vi "一体站流程质控自动启动.vi"(6 "CODMn量程切换":enum32{"H", "L", "AUTO"}(ring)=enum."AUTO", 8 "总磷量程切换":enum32{"H", "L", "AUTO"}(ring)=enum."AUTO", 9 "总氮量程切换":enum32{"H", "L", "AUTO"}(ring)=enum."AUTO", 10 "氨氮量程切换":enum32{"H", "L", "AUTO"}(ring)=enum."AUTO", 11 "参数":T1={"是否启用仪器"=FALSE, "CODMn"={"启动测量模式"={"测量模式"=enum."水样测量"}, "确定按钮"=TRUE}, "启动模块"={"氨氮"=FALSE, "总磷"=FALSE, "总氮"=FALSE, "CODMn"=FALSE, "CODCr"=FALSE}, "常规启动"=FALSE, "直接启动"=FALSE}) -> ()   [LabVIEW 2016, in "质控单元.lvlib"]
panel:
  out "枚举 2":enum16{"初始化", "采配水启动", "等待", "配水", "排水", "结束"}(ring)
  out "枚举":enum16{"初始化", "采配水启动", "等待", "配水", "排水", "结束"}(ring)
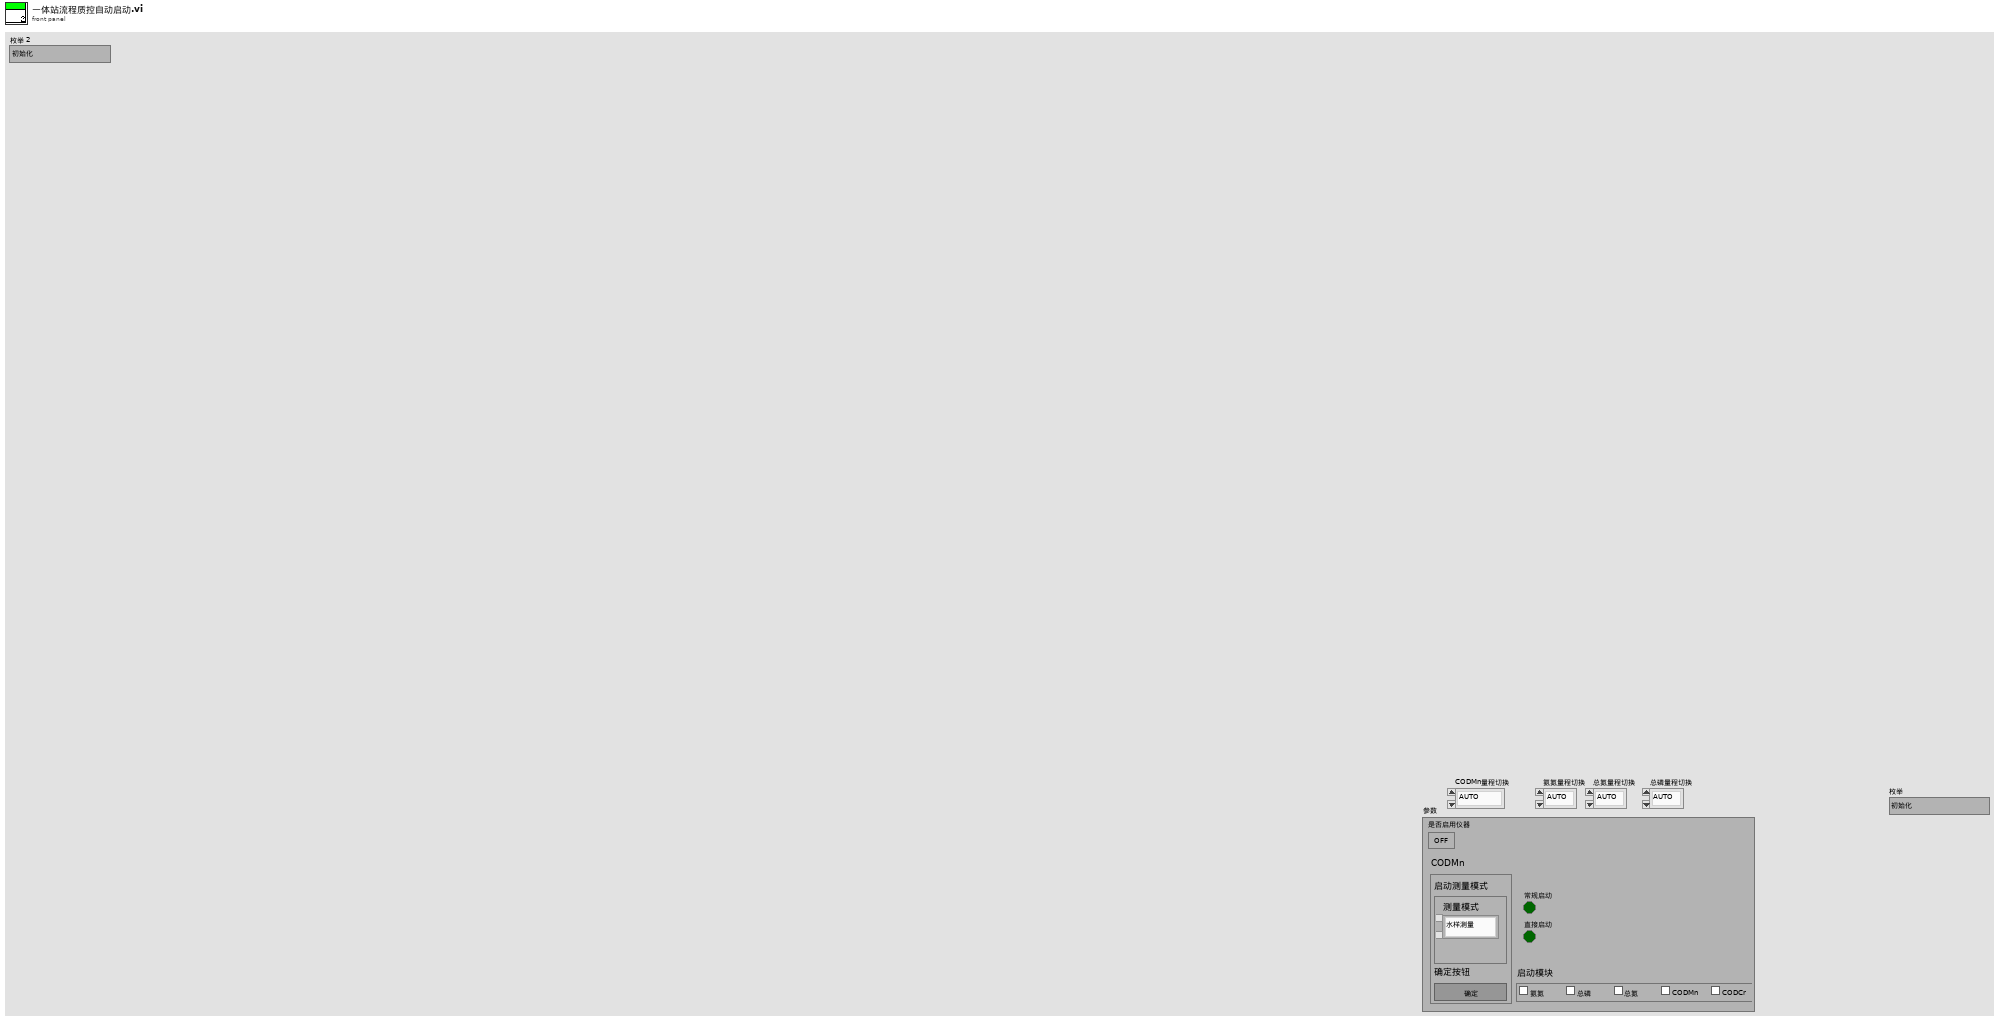
[diagram p1: front panel]
types:
  T1 = cluster{"是否启用仪器":bool, "CODMn":cluster{"启动测量模式":cluster{"测量模式":enum16{"水样测量", "标样核查", "加标回收", "平行样", "校零", "校标"}}, "确定按钮":bool}, "启动模块":cluster{"氨氮":bool, "总磷":bool, "总氮":bool, "CODMn":bool, "CODCr":bool}, "常规启动":bool, "直接启动":bool}
  T2 = cluster{"命令":string, cluster{"starting address":u16, "holding register value":u16}}
  T3 = cluster{"R0":i16, "R1":i16, "R2":i16, "R3":i16, "R4":i16, "R5":i16, "R6":i16, "R7":i16, "R8":i16, "R9":i16, "R10":i16, "R11":i16, "R12":i16, "R13":i16, "R14":i16, "R15":i16, "R16":i16, "R17":i16, "R18":i16, "R19":i16, "R20":i16, "R21":i16, "R22":i16, "R23":i16, "R24":i16, "R25":i16, "R26":i16, "R27":i16, "R28":i16, "R29":i16, "R30":i16, "R31":i16, "R32":i16, "R33":i16, "R34":i16, "R35":i16, "R36":i16, "R37":i16, "R38":i16, "R39":i16, "R40":i16, "R41":i16, "R42":i16, "R43":i16, "R44":i16, "R45":i16, "R46":i16, "R47":i16, "R48":i16, "R49":i16, "R50":i16, "R51":i16, "R52":i16, "R53":i16, "R54":i16, "R55":i16, "R56":i16}
  T4 = enum32{"Bad", "Idle", "Run top level", "Running"}
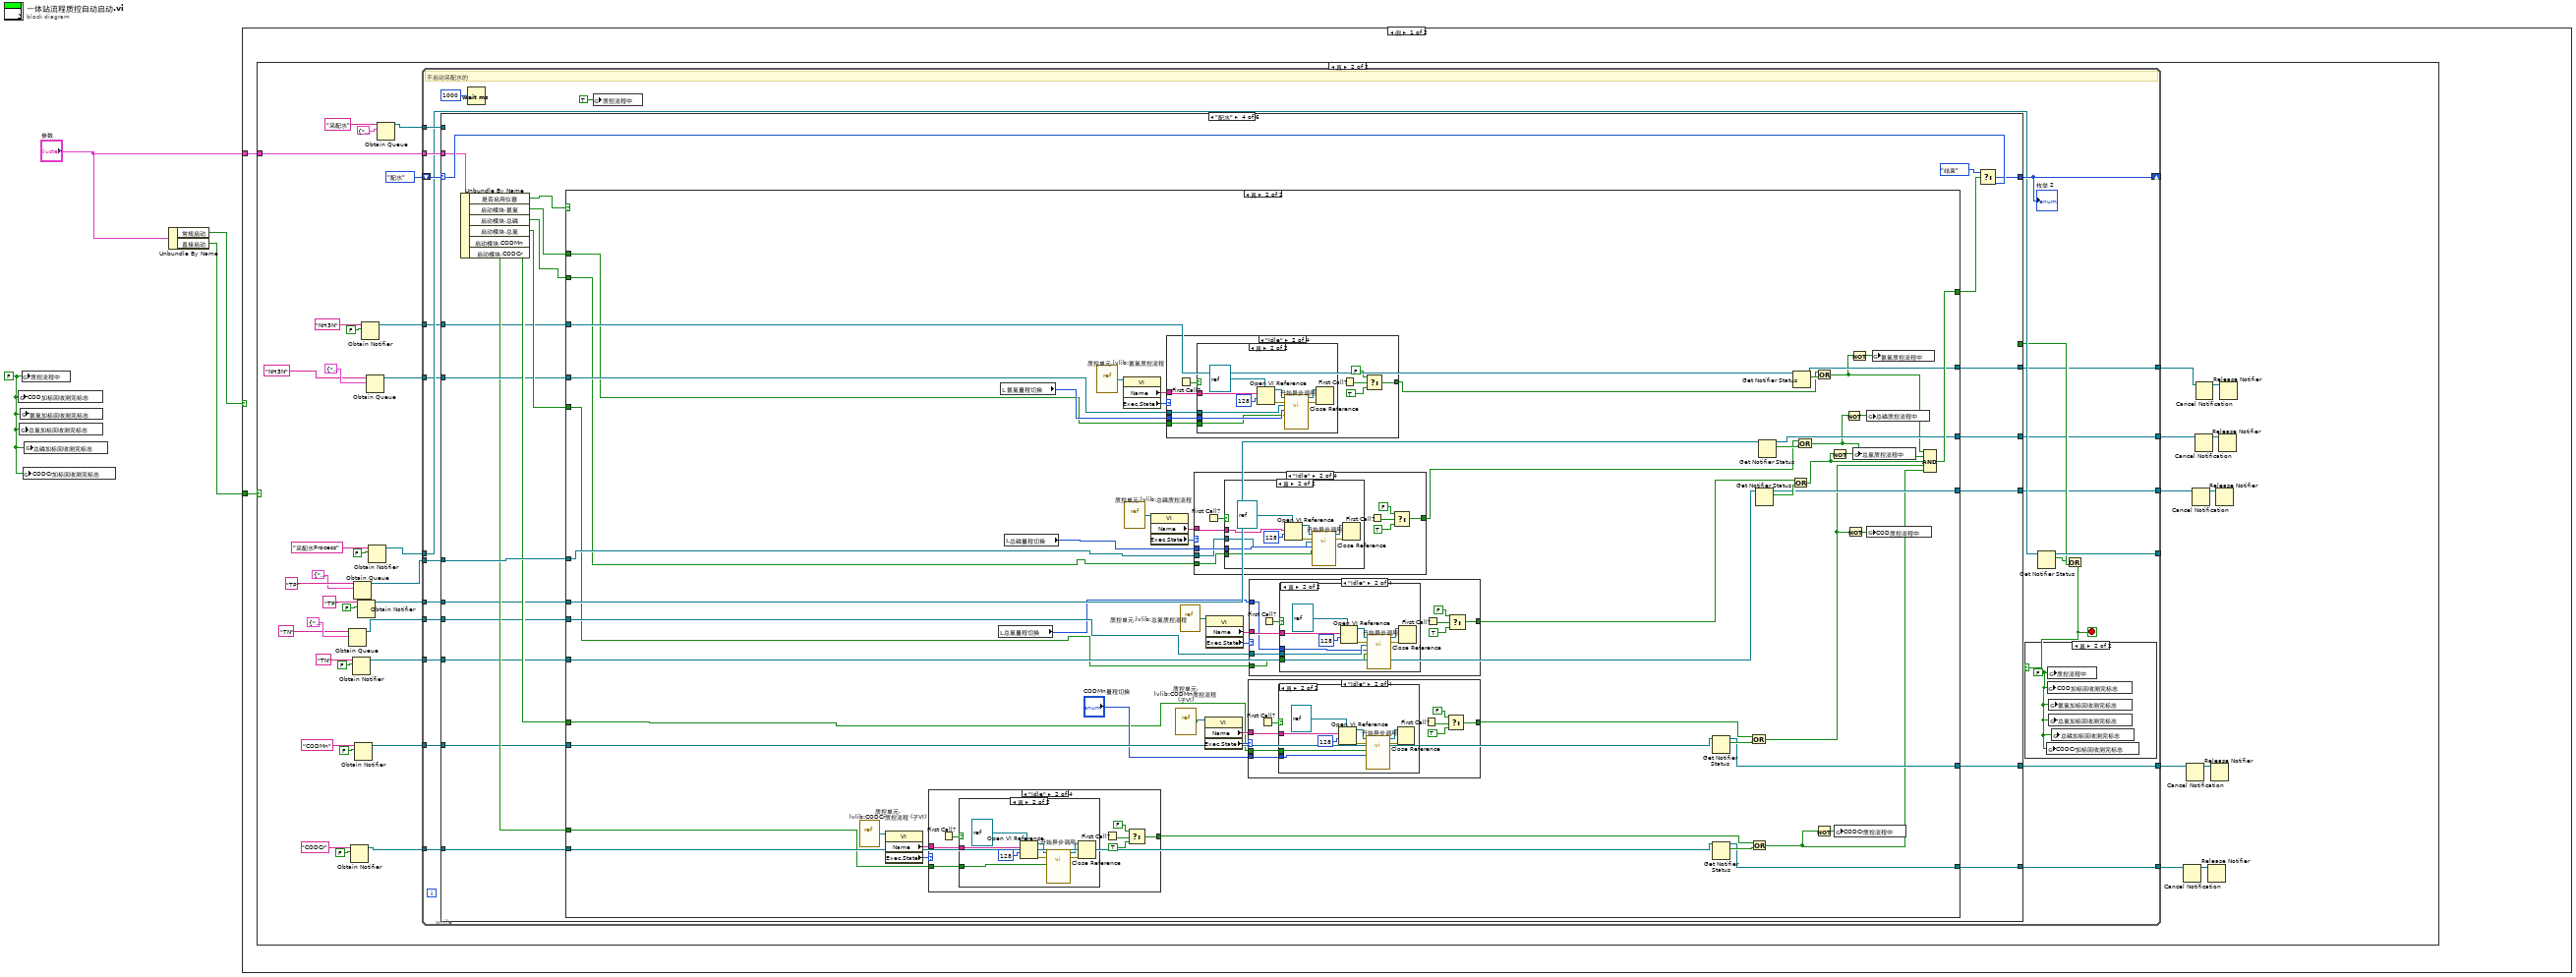
[diagram p0: block diagram]
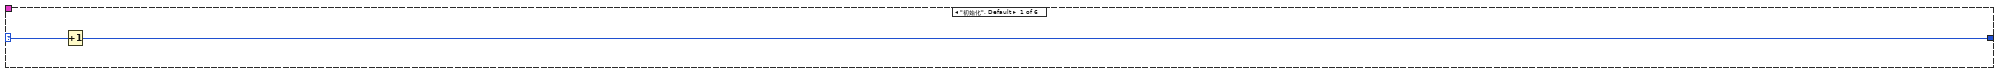
[diagram p4: hidden frame]
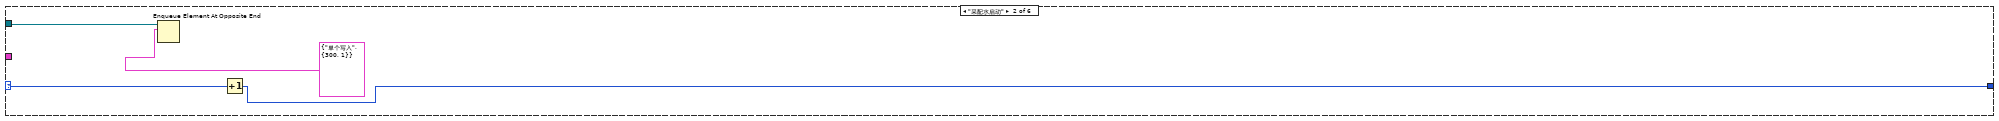
[diagram p5: hidden frame]
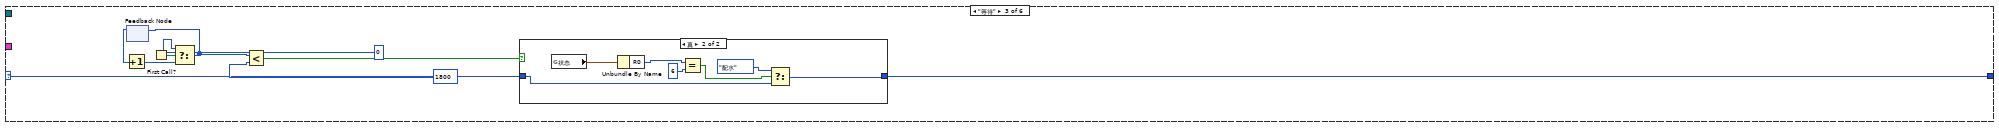
[diagram p6: hidden frame]
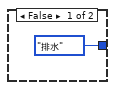
[diagram p7: hidden frame]
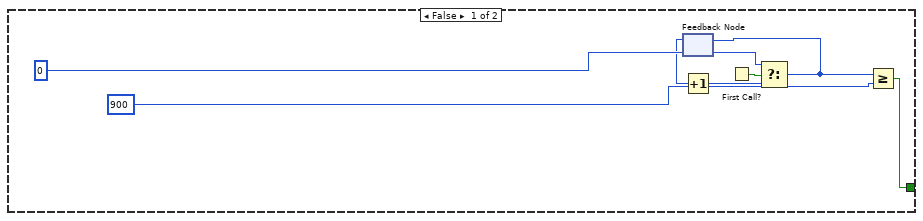
[diagram p8: hidden frame]
diagram:
  w1 = FALSE ("质控流程中")
  n1 = global write "质控测完标志全局 1.vi" "COD加标回收测完标志"(w1) -> ()
  n2 = global write "质控测完标志全局 1.vi" "总氮加标回收测完标志"(w1) -> ()
  n3 = global write "质控测完标志全局 1.vi" "氨氮加标回收测完标志"(w1) -> ()
  n4 = global write "质控测完标志全局 1.vi" "质控流程中"(w1) -> ()
  n5 = global write "质控测完标志全局 1.vi" "CODCr加标回收测完标志"(w1) -> ()
  n6 = global write "质控测完标志全局 1.vi" "总磷加标回收测完标志"(w1) -> ()
  n7 = Unbundle By Name("参数") -> ("常规启动"=w3:bool, "直接启动"=w2:bool)
  n8 = case shown="假" w3 {
    tunnel: "参数" -> [w5 w313]
    tunnel: w2 -> [w6 _]
    frame False {
      n9 = case shown="真" w6 {
        tunnel: w5 -> [_ w47]
        frame False {
        }
        frame True {
          n10 = Obtain Queue(name (unnamed)="TN" ("名称（未命名）"), element data type=cluster{"命令":string, "data":variant} {"命令"="", "data"=variant}) -> (queue out=w32:refnum<queue>)  [unwired: 3 in, 2 out]
          n11 = Obtain Notifier(name (unnamed)="CODCr" ("名称（未命名）"), notification data type=FALSE) -> (notifier out=w9:refnum<notifier>)  [unwired: 2 in, 2 out]
          n12 = Obtain Notifier(name (unnamed)="TN" ("名称（未命名）"), notification data type=FALSE) -> (notifier out=w15:refnum<notifier>)  [unwired: 2 in, 2 out]
          n13 = Obtain Queue(name (unnamed)="TP" ("名称（未命名）"), element data type=cluster{"命令":string, "data":variant} {"命令"="", "data"=variant}) -> (queue out=w38:refnum<queue>)  [unwired: 3 in, 2 out]
          n14 = Obtain Notifier(name (unnamed)="CODMn" ("名称（未命名）"), notification data type=FALSE) -> (notifier out=w12:refnum<notifier>)  [unwired: 2 in, 2 out]
          n15 = Obtain Notifier(name (unnamed)="TP" ("名称（未命名）"), notification data type=FALSE) -> (notifier out=w18:refnum<notifier>)  [unwired: 2 in, 2 out]
          n16 = Obtain Notifier(name (unnamed)="NH3N" ("名称（未命名）"), notification data type=FALSE) -> (notifier out=w21:refnum<notifier>)  [unwired: 2 in, 2 out]
          n17 = Obtain Queue(name (unnamed)="NH3N" ("名称（未命名）"), element data type=cluster{"命令":string, "data":variant} {"命令"="", "data"=variant}) -> (queue out=w35:refnum<queue>)  [unwired: 3 in, 2 out]
          n18 = Obtain Notifier(name (unnamed)="采配水Process" ("名称（未命名）"), notification data type=FALSE) -> (notifier out=w41:refnum<notifier>)  [unwired: 2 in, 2 out]
          n19 = Obtain Queue(name (unnamed)="采配水" ("名称（未命名）"), element data type=cluster{"命令":string, "数据":variant} {"命令"="", "数据"=variant}) -> (queue out=w44:refnum<queue>)  [unwired: 3 in, 2 out]
          n20 = while {
            tunnel: w44 -> [w72]
            shift-right: [w70] -> _
            shift-left: enum16{"初始化", "采配水启动", "等待", "配水", "排水", "结束"}."配水" ("枚举") -> [w71]
            tunnel: w38 -> [w68]
            tunnel: w47 -> [w67]
            tunnel: w41 -> [w66]
            tunnel: [w65] -> _
            tunnel: w35 -> [w62]
            tunnel: w32 -> [w59]
            tunnel: w21 -> [w58]
            tunnel: [w57] -> w19
            tunnel: w18 -> [w56]
            tunnel: [w55] -> w16
            tunnel: w15 -> [w54]
            tunnel: [w53] -> w13
            tunnel: w12 -> [w52]
            tunnel: [w51] -> w10
            tunnel: w9 -> [w50]
            tunnel: [w49] -> w7
            stop <- w61 stop-if-true
            # "不启动采配水的"
            n21 = case shown="\"配水\"" w71 {
              selector: w71 -> [w75 w77 w86 w119 w276 w281]
              tunnel: w72 -> [_ w78 _ _ w277 _]
              tunnel: [w74 w76 w85 w118 w275 w280] -> w70
              tunnel: [_ _ _ _ _ TRUE] -> w64
              tunnel: w68 -> [_ _ _ w117 _ _]
              tunnel: w67 -> [_ _ _ w114 _ _]
              tunnel: w62 -> [_ _ _ w109 _ _]
              tunnel: w59 -> [_ _ _ w107 _ _]
              tunnel: w58 -> [_ _ _ w106 _ _]
              tunnel: [_ _ _ w105 _ _] -> w57
              tunnel: w56 -> [_ _ _ w104 _ _]
              tunnel: [_ _ _ w103 _ _] -> w55
              tunnel: w54 -> [_ _ _ w102 _ _]
              tunnel: [_ _ _ w101 _ _] -> w53
              tunnel: w52 -> [_ _ _ w100 _ _]
              tunnel: [_ _ _ w99 _ _] -> w51
              tunnel: w50 -> [_ _ _ w98 _ _]
              tunnel: [_ _ _ w97 _ _] -> w49
              frame "初始化", Default {
                n22 = Increment(x=w75) -> (x+1=w74:enum16{"初始化", "采配水启动", "等待", "配水", "排水", "结束"})
              }
              frame "采配水启动" {
                n23 = Enqueue Element At Opposite End(queue=w78, element=T2 {"命令"="单个写入", {"starting address"=300, "holding register value"=1}} ("元素")) -> ()  [unwired: 2 in, 3 out]
                n24 = Increment(x=w77) -> (x+1=w76:enum16{"初始化", "采配水启动", "等待", "配水", "排水", "结束"})
              }
              frame "等待" {
                n25 = feedback #1() -> (w82:i32)  [unwired: 1 in]
                n26 = Increment(x=w82) -> (x+1=w81:i32)
                n27 = First Call?() -> (First Call?: T/F=w83:bool)
                n28 = Select(t=0, s=w83, f=w81) -> (s? t:f=w80:i32)
                n29 = feedback-in #1(w80) -> ()
                n30 = Less?(x=w80, y=1800) -> (x < y?=w87:bool)
                n31 = case shown="真" w87 {
                  tunnel: w86 -> [_ w92]
                  tunnel: [enum16{"初始化", "采配水启动", "等待", "配水", "排水", "结束"}."排水" ("枚举") w91] -> w85
                  frame False {
                  }
                  frame True {
                    n32 = global read "与采配水交互全局.vi" "状态"() -> (w90:T3)
                    n33 = Unbundle By Name(w90) -> ("R0"=w96:i16)
                    n34 = Equal?(x=w96, y=i16 6) -> (x = y?=w94:bool)
                    n35 = Select(t=enum16{"初始化", "采配水启动", "等待", "配水", "排水", "结束"}."配水" ("枚举"), s=w94, f=w92) -> (s? t:f=w91:enum16{"初始化", "采配水启动", "等待", "配水", "排水", "结束"})
                  }
                }
              }
              frame "配水" {
                n36 = Unbundle By Name(w114) -> ("是否启用仪器"=w116:bool, "启动模块.氨氮"=w112:bool, "启动模块.总磷"=w113:bool, "启动模块.总氮"=w110:bool, "启动模块.CODMn"=w111:bool, "启动模块.CODCr"=w108:bool)
                n37 = case shown="真" w116 {
                  tunnel: w117 -> [_ w149]
                  tunnel: [w121 w185] -> w115
                  tunnel: w113 -> [_ w147]
                  tunnel: w112 -> [_ w154]
                  tunnel: w111 -> [_ w136]
                  tunnel: w110 -> [_ w141]
                  tunnel: w109 -> [_ w156]
                  tunnel: w108 -> [_ w129]
                  tunnel: w107 -> [_ w143]
                  tunnel: w106 -> [_ w183]
                  tunnel: [_ w182] -> w105
                  tunnel: w104 -> [_ w180]
                  tunnel: [_ w179] -> w103
                  tunnel: w102 -> [_ w177]
                  tunnel: [_ w176] -> w101
                  tunnel: w100 -> [_ w174]
                  tunnel: [_ w173] -> w99
                  tunnel: w98 -> [_ w171]
                  tunnel: [_ w170] -> w97
                  frame False {
                    n38 = feedback #2() -> (w125:i32)  [unwired: 1 in]
                    n39 = Increment(x=w125) -> (x+1=w124:i32)
                    n40 = First Call?() -> (First Call?: T/F=w126:bool)
                    n41 = Select(t=0, s=w126, f=w124) -> (s? t:f=w122:i32)
                    n42 = feedback-in #2(w122) -> ()
                    n43 = Greater Or Equal?(x=w122, y=900) -> (x >= y?=w121:bool)
                  }
                  frame True {
                    n44 = vi-ref "质控单元.lvlib:CODCr质控流程 (子VI).vi"() -> (w131:refnum<vi>)
                    n45 = property class="VI"(reference=w131) -> ("Name"=w132:string, "Exec.State"=w130:T4)  [unwired: 1 in, 2 out]
                    n46 = case shown="\"Idle\"" w130 {
                      tunnel: w132 -> [_ w192 _ _]
                      tunnel: [_ w187 _ _] -> w128
                      tunnel: w129 -> [_ w186 _ _]
                      frame "Bad", Default {
                      }
                      frame "Idle" {
                        n47 = First Call?() -> (First Call?: T/F=w191:bool)
                        n48 = case shown="真" w191 {
                          tunnel: w192 -> [_ w199]
                          tunnel: w186 -> [_ w193]
                          frame False {
                          }
                          frame True {
                            n49 = Open VI Reference(type specifier VI Refnum (for type only)=refnum<vi> refnum ("类型说明符VI引用句柄（仅用于类型）"), vi path=w199, options=128 ("选项")) -> (vi reference=w200:refnum<vi>, error out=w196:errorcluster)  [unwired: 3 in]
                            n50 = call-by-ref "开始异步调用"(reference=w200, error in=w196, "CODCr"=w193) -> (reference out=w198:refnum<vi>, error out=w197:errorcluster)  [unwired: 9 in, 1 out]
                            n51 = Close Reference(reference=w198, error in (no error)=w197) -> ()  [unwired: 1 out]
                          }
                        }
                        n52 = First Call?() -> (First Call?: T/F=w190:bool)
                        n53 = Select(t=FALSE, s=w190, f=TRUE) -> (s? t:f=w187:bool)
                      }
                      frame "Run top level" {
                      }
                      frame "Running" {
                      }
                    }
                    n54 = local read "总氮量程切换"() -> (w142:enum32{"H", "L", "AUTO"})
                    n55 = local read "氨氮量程切换"() -> (w155:enum32{"H", "L", "AUTO"})
                    n56 = local read "总磷量程切换"() -> (w148:enum32{"H", "L", "AUTO"})
                    n57 = vi-ref "质控单元.lvlib:氨氮质控流程.vi"() -> (w158:refnum<vi>)
                    n58 = property class="VI"(reference=w158) -> ("Name"=w159:string, "Exec.State"=w157:T4)  [unwired: 1 in, 2 out]
                    n59 = vi-ref "质控单元.lvlib:总磷质控流程.vi"() -> (w151:refnum<vi>)
                    n60 = property class="VI"(reference=w151) -> ("Name"=w150:string, "Exec.State"=w152:T4)  [unwired: 1 in, 2 out]
                    n61 = case shown="\"Idle\"" w157 {
                      tunnel: w159 -> [_ w264 _ _]
                      tunnel: [_ w259 _ _] -> w153
                      tunnel: w156 -> [_ w258 _ _]
                      tunnel: w155 -> [_ w257 _ _]
                      tunnel: w154 -> [_ w256 _ _]
                      frame "Bad", Default {
                      }
                      frame "Idle" {
                        n62 = First Call?() -> (First Call?: T/F=w263:bool)
                        n63 = case shown="真" w263 {
                          tunnel: w264 -> [_ w273]
                          tunnel: w258 -> [_ w267]
                          tunnel: w257 -> [_ w266]
                          tunnel: w256 -> [_ w265]
                          frame False {
                          }
                          frame True {
                            n64 = Open VI Reference(type specifier VI Refnum (for type only)=refnum<vi> refnum ("类型说明符VI引用句柄（仅用于类型）"), vi path=w273, options=128 ("选项")) -> (vi reference=w274:refnum<vi>, error out=w270:errorcluster)  [unwired: 3 in]
                            n65 = call-by-ref "开始异步调用"(reference=w274, error in=w270, "队列输入NH3"=w267, "氨氮"=w265, "氨氮量程切换"=w266) -> (reference out=w272:refnum<vi>, error out=w271:errorcluster)  [unwired: 7 in, 1 out]
                            n66 = Close Reference(reference=w272, error in (no error)=w271) -> ()  [unwired: 1 out]
                          }
                        }
                        n67 = First Call?() -> (First Call?: T/F=w262:bool)
                        n68 = Select(t=FALSE, s=w262, f=TRUE) -> (s? t:f=w259:bool)
                      }
                      frame "Run top level" {
                      }
                      frame "Running" {
                      }
                    }
                    n69 = vi-ref "质控单元.lvlib:CODMn质控流程 (子VI).vi"() -> (w139:refnum<vi>)
                    n70 = vi-ref "质控单元.lvlib:总氮质控流程.vi"() -> (w145:refnum<vi>)
                    n71 = case shown="\"Idle\"" w152 {
                      tunnel: w150 -> [_ w245 _ _]
                      tunnel: [_ w240 _ _] -> w134
                      tunnel: w148 -> [_ w239 _ _]
                      tunnel: w147 -> [_ w238 _ _]
                      tunnel: w149 -> [_ w237 _ _]
                      frame "Bad", Default {
                      }
                      frame "Idle" {
                        n72 = First Call?() -> (First Call?: T/F=w244:bool)
                        n73 = case shown="真" w244 {
                          tunnel: w245 -> [_ w246]
                          tunnel: w239 -> [_ w254]
                          tunnel: w238 -> [_ w252]
                          tunnel: w237 -> [_ w251]
                          frame False {
                          }
                          frame True {
                            n74 = Open VI Reference(type specifier VI Refnum (for type only)=refnum<vi> refnum ("类型说明符VI引用句柄（仅用于类型）"), vi path=w246, options=128 ("选项")) -> (vi reference=w250:refnum<vi>, error out=w249:errorcluster)  [unwired: 3 in]
                            n75 = call-by-ref "开始异步调用"(reference=w250, error in=w249, "队列输入TP"=w251, "总磷"=w252, "总磷量程切换"=w254) -> (reference out=w248:refnum<vi>, error out=w247:errorcluster)  [unwired: 7 in, 1 out]
                            n76 = Close Reference(reference=w248, error in (no error)=w247) -> ()  [unwired: 1 out]
                          }
                        }
                        n77 = First Call?() -> (First Call?: T/F=w243:bool)
                        n78 = Select(t=FALSE, s=w243, f=TRUE) -> (s? t:f=w240:bool)
                      }
                      frame "Run top level" {
                      }
                      frame "Running" {
                      }
                    }
                    n79 = property class="VI"(reference=w139) -> ("Name"=w138:string, "Exec.State"=w140:T4)  [unwired: 1 in, 2 out]
                    n80 = property class="VI"(reference=w145) -> ("Name"=w146:string, "Exec.State"=w144:T4)  [unwired: 1 in, 2 out]
                    n81 = case shown="\"Idle\"" w140 {
                      tunnel: w138 -> [_ w208 _ _]
                      tunnel: [_ w203 _ _] -> w135
                      tunnel: w136 -> [_ w202 _ _]
                      tunnel: "CODMn量程切换" -> [_ w201 _ _]
                      frame "Bad", Default {
                      }
                      frame "Idle" {
                        n82 = First Call?() -> (First Call?: T/F=w207:bool)
                        n83 = case shown="真" w207 {
                          tunnel: w208 -> [_ w216]
                          tunnel: w202 -> [_ w210]
                          tunnel: w201 -> [_ w209]
                          frame False {
                          }
                          frame True {
                            n84 = Open VI Reference(type specifier VI Refnum (for type only)=refnum<vi> refnum ("类型说明符VI引用句柄（仅用于类型）"), vi path=w216, options=128 ("选项")) -> (vi reference=w217:refnum<vi>, error out=w213:errorcluster)  [unwired: 3 in]
                            n85 = call-by-ref "开始异步调用"(reference=w217, error in=w213, "CODMn量程切换"=w209, "CODMn"=w210) -> (reference out=w215:refnum<vi>, error out=w214:errorcluster)  [unwired: 8 in, 1 out]
                            n86 = Close Reference(reference=w215, error in (no error)=w214) -> ()  [unwired: 1 out]
                          }
                        }
                        n87 = First Call?() -> (First Call?: T/F=w206:bool)
                        n88 = Select(t=FALSE, s=w206, f=TRUE) -> (s? t:f=w203:bool)
                      }
                      frame "Run top level" {
                      }
                      frame "Running" {
                      }
                    }
                    n89 = case shown="\"Idle\"" w144 {
                      tunnel: w146 -> [_ w226 _ _]
                      tunnel: [_ w221 _ _] -> w133
                      tunnel: w143 -> [_ w220 _ _]
                      tunnel: w142 -> [_ w219 _ _]
                      tunnel: w141 -> [_ w218 _ _]
                      frame "Bad", Default {
                      }
                      frame "Idle" {
                        n90 = First Call?() -> (First Call?: T/F=w225:bool)
                        n91 = case shown="真" w225 {
                          tunnel: w226 -> [_ w236]
                          tunnel: w220 -> [_ w229]
                          tunnel: w219 -> [_ w228]
                          tunnel: w218 -> [_ w227]
                          frame False {
                          }
                          frame True {
                            n92 = Open VI Reference(type specifier VI Refnum (for type only)=refnum<vi> refnum ("类型说明符VI引用句柄（仅用于类型）"), vi path=w236, options=128 ("选项")) -> (vi reference=w231:refnum<vi>, error out=w230:errorcluster)  [unwired: 3 in]
                            n93 = call-by-ref "开始异步调用"(reference=w231, error in=w230, "队列输入TN"=w229, "总氮"=w227, "总氮量程切换"=w228) -> (reference out=w235:refnum<vi>, error out=w234:errorcluster)  [unwired: 7 in, 1 out]
                            n94 = Close Reference(reference=w235, error in (no error)=w234) -> ()  [unwired: 1 out]
                          }
                        }
                        n95 = First Call?() -> (First Call?: T/F=w224:bool)
                        n96 = Select(t=FALSE, s=w224, f=TRUE) -> (s? t:f=w221:bool)
                      }
                      frame "Run top level" {
                      }
                      frame "Running" {
                      }
                    }
                    n97 = Get Notifier Status(notifier=w174) -> (notifier out=w173:refnum<notifier>, current notification=w175:bool)  [unwired: 1 in, 3 out]
                    n98 = Get Notifier Status(notifier=w171) -> (notifier out=w170:refnum<notifier>, current notification=w172:bool)  [unwired: 1 in, 3 out]
                    n99 = Or(x=w135, y=w175) -> (x .or. y?=w162:bool)
                    n100 = Or(x=w128, y=w172) -> (x .or. y?=w160:bool)
                    n101 = Get Notifier Status(notifier=w177) -> (notifier out=w176:refnum<notifier>, current notification=w178:bool)  [unwired: 1 in, 3 out]
                    n102 = Get Notifier Status(notifier=w180) -> (notifier out=w179:refnum<notifier>, current notification=w181:bool)  [unwired: 1 in, 3 out]
                    n103 = Or(x=w133, y=w178) -> (x .or. y?=w164:bool)
                    n104 = Get Notifier Status(notifier=w183) -> (notifier out=w182:refnum<notifier>, current notification=w184:bool)  [unwired: 1 in, 3 out]
                    n105 = Or(x=w134, y=w181) -> (x .or. y?=w166:bool)
                    n106 = Not(x=w160) -> (.not. x?=w161:bool)
                    n107 = Or(x=w153, y=w184) -> (x .or. y?=w168:bool)
                    n108 = Not(x=w164) -> (.not. x?=w165:bool)
                    n109 = global write "质控测完标志全局 1.vi" "CODCr质控流程中"(w161) -> ()
                    n110 = Not(x=w166) -> (.not. x?=w167:bool)
                    n111 = Not(x=w162) -> (.not. x?=w163:bool)
                    n112 = Not(x=w168) -> (.not. x?=w169:bool)
                    n113 = global write "质控测完标志全局 1.vi" "总氮质控流程中"(w165) -> ()
                    n114 = global write "质控测完标志全局 1.vi" "总磷质控流程中"(w167) -> ()
                    n115 = global write "质控测完标志全局 1.vi" "COD质控流程中"(w163) -> ()
                    n116 = global write "质控测完标志全局 1.vi" "氨氮质控流程中"(w169) -> ()
                    n117 = Compound Arithmetic op=AND ("复合运算")(w168, w166, w164, w162, w160) -> (w185:bool)
                  }
                }
                n118 = Select(t=enum16{"初始化", "采配水启动", "等待", "配水", "排水", "结束"}."结束" ("枚举"), s=w115, f=w119) -> (s? t:f=w118:enum16{"初始化", "采配水启动", "等待", "配水", "排水", "结束"})
              }
              frame "排水" {
                n119 = Enqueue Element At Opposite End(queue=w277, element=T2 {"命令"="单个写入", {"starting address"=303, "holding register value"=1}} ("元素")) -> ()  [unwired: 2 in, 3 out]
                n120 = Increment(x=w276) -> (x+1=w275:enum16{"初始化", "采配水启动", "等待", "配水", "排水", "结束"})
              }
              frame "结束" {
                n121 = Increment(x=w281) -> (x+1=w280:enum16{"初始化", "采配水启动", "等待", "配水", "排水", "结束"})
              }
            }
            "枚举 2" <- w70
            n122 = Wait (ms)(milliseconds to wait=u32 1000 ("等待时间（毫秒）")) -> ()  [unwired: 1 out]
            n123 = global write "质控测完标志全局 1.vi" "质控流程中"(TRUE ("质控流程中")) -> ()
            n124 = Get Notifier Status(notifier=w66) -> (notifier out=w65:refnum<notifier>, current notification=w63:bool)  [unwired: 1 in, 3 out]
            n125 = Or(x=w63, y=w64) -> (x .or. y?=w61:bool)
            n126 = case shown="真" w61 {
              frame False {
              }
              frame True {
                w73 = FALSE ("质控流程中")
                n127 = global write "质控测完标志全局 1.vi" "CODCr加标回收测完标志"(w73) -> ()
                n128 = global write "质控测完标志全局 1.vi" "COD加标回收测完标志"(w73) -> ()
                n129 = global write "质控测完标志全局 1.vi" "质控流程中"(w73) -> ()
                n130 = global write "质控测完标志全局 1.vi" "总氮加标回收测完标志"(w73) -> ()
                n131 = global write "质控测完标志全局 1.vi" "氨氮加标回收测完标志"(w73) -> ()
                n132 = global write "质控测完标志全局 1.vi" "总磷加标回收测完标志"(w73) -> ()
              }
            }
          }
          n133 = Cancel Notification(0:w7) -> (8:w8:refnum<notifier>)  [unwired: 1 in, 2 out]
          n134 = Cancel Notification(0:w10) -> (8:w11:refnum<notifier>)  [unwired: 1 in, 2 out]
          n135 = Cancel Notification(0:w13) -> (8:w14:refnum<notifier>)  [unwired: 1 in, 2 out]
          n136 = Cancel Notification(0:w16) -> (8:w17:refnum<notifier>)  [unwired: 1 in, 2 out]
          n137 = Cancel Notification(0:w19) -> (8:w20:refnum<notifier>)  [unwired: 1 in, 2 out]
          n138 = Release Notifier(notifier=w8) -> ()  [unwired: 2 in, 3 out]
          n139 = Release Notifier(notifier=w11) -> ()  [unwired: 2 in, 3 out]
          n140 = Release Notifier(notifier=w14) -> ()  [unwired: 2 in, 3 out]
          n141 = Release Notifier(notifier=w17) -> ()  [unwired: 2 in, 3 out]
          n142 = Release Notifier(notifier=w20) -> ()  [unwired: 2 in, 3 out]
        }
      }
    }
    frame True {
      n143 = Obtain Notifier(name (unnamed)="采配水Process" ("名称（未命名）"), notification data type=FALSE) -> (notifier out=w316:refnum<notifier>)  [unwired: 2 in, 2 out]
      n144 = Obtain Notifier(name (unnamed)="TN" ("名称（未命名）"), notification data type=FALSE) -> (notifier out=w298:refnum<notifier>)  [unwired: 2 in, 2 out]
      n145 = Obtain Notifier(name (unnamed)="CODCr" ("名称（未命名）"), notification data type=FALSE) -> (notifier out=w292:refnum<notifier>)  [unwired: 2 in, 2 out]
      n146 = Obtain Queue(name (unnamed)="TN" ("名称（未命名）"), element data type=cluster{"命令":string, "data":variant} {"命令"="", "data"=variant}) -> (queue out=w310:refnum<queue>)  [unwired: 3 in, 2 out]
      n147 = Obtain Notifier(name (unnamed)="CODMn" ("名称（未命名）"), notification data type=FALSE) -> (notifier out=w293:refnum<notifier>)  [unwired: 2 in, 2 out]
      n148 = Obtain Notifier(name (unnamed)="TP" ("名称（未命名）"), notification data type=FALSE) -> (notifier out=w299:refnum<notifier>)  [unwired: 2 in, 2 out]
      n149 = Obtain Queue(name (unnamed)="TP" ("名称（未命名）"), element data type=cluster{"命令":string, "data":variant} {"命令"="", "data"=variant}) -> (queue out=w319:refnum<queue>)  [unwired: 3 in, 2 out]
      n150 = Obtain Queue(name (unnamed)="NH3N" ("名称（未命名）"), element data type=cluster{"命令":string, "data":variant} {"命令"="", "data"=variant}) -> (queue out=w305:refnum<queue>)  [unwired: 3 in, 2 out]
      n151 = Obtain Notifier(name (unnamed)="NH3N" ("名称（未命名）"), notification data type=FALSE) -> (notifier out=w304:refnum<notifier>)  [unwired: 2 in, 2 out]
      n152 = Obtain Queue(name (unnamed)="采配水" ("名称（未命名）"), element data type=cluster{"命令":string, "数据":variant} {"命令"="", "数据"=variant}) -> (queue out=w323:refnum<queue>)  [unwired: 3 in, 2 out]
      n153 = while {
        tunnel: w323 -> [w349]
        shift-right: [w347] -> _
        shift-left: enum16{"初始化", "采配水启动", "等待", "配水", "排水", "结束"}."初始化" ("枚举") -> [w348]
        tunnel: w319 -> [w345]
        tunnel: w313 -> [w344]
        tunnel: w316 -> [w343]
        tunnel: [w342] -> w315
        tunnel: w310 -> [w337]
        tunnel: w305 -> [w336]
        tunnel: w304 -> [w335]
        tunnel: w299 -> [w334]
        tunnel: w298 -> [w333]
        tunnel: w293 -> [w332]
        tunnel: w292 -> [w331]
        tunnel: [w330] -> w290
        tunnel: [w329] -> w288
        tunnel: [w328] -> w286
        tunnel: [w327] -> w284
        tunnel: [w326] -> w282
        stop <- w339 stop-if-true
        # "启动采配水的"
        n154 = case shown="\"配水\"" w348 {
          selector: w348 -> [w352 w354 w363 w396 w548 w553]
          tunnel: w349 -> [_ w355 _ _ w549 _]
          tunnel: [w351 w353 w362 w395 w547 w552] -> w347
          tunnel: [_ _ _ _ _ TRUE] -> w341
          tunnel: w345 -> [_ _ _ w394 _ _]
          tunnel: w344 -> [_ _ _ w391 _ _]
          tunnel: w337 -> [_ _ _ w385 _ _]
          tunnel: w336 -> [_ _ _ w384 _ _]
          tunnel: w335 -> [_ _ _ w383 _ _]
          tunnel: w334 -> [_ _ _ w382 _ _]
          tunnel: w333 -> [_ _ _ w381 _ _]
          tunnel: w332 -> [_ _ _ w380 _ _]
          tunnel: w331 -> [_ _ _ w379 _ _]
          tunnel: [_ _ _ w378 _ _] -> w330
          tunnel: [_ _ _ w377 _ _] -> w329
          tunnel: [_ _ _ w376 _ _] -> w328
          tunnel: [_ _ _ w375 _ _] -> w327
          tunnel: [_ _ _ w374 _ _] -> w326
          frame "初始化", Default {
            n155 = Increment(x=w352) -> (x+1=w351:enum16{"初始化", "采配水启动", "等待", "配水", "排水", "结束"})
          }
          frame "采配水启动" {
            n156 = Enqueue Element At Opposite End(queue=w355, element=T2 {"命令"="单个写入", {"starting address"=300, "holding register value"=3}} ("元素")) -> ()  [unwired: 2 in, 3 out]
            n157 = Increment(x=w354) -> (x+1=w353:enum16{"初始化", "采配水启动", "等待", "配水", "排水", "结束"})
          }
          frame "等待" {
            n158 = feedback #3() -> (w359:i32)  [unwired: 1 in]
            n159 = Increment(x=w359) -> (x+1=w358:i32)
            n160 = First Call?() -> (First Call?: T/F=w360:bool)
            n161 = Select(t=0, s=w360, f=w358) -> (s? t:f=w357:i32)
            n162 = feedback-in #3(w357) -> ()
            n163 = Less?(x=w357, y=1800) -> (x < y?=w364:bool)
            n164 = case shown="真" w364 {
              tunnel: w363 -> [_ w369]
              tunnel: [enum16{"初始化", "采配水启动", "等待", "配水", "排水", "结束"}."排水" ("枚举") w368] -> w362
              frame False {
              }
              frame True {
                n165 = global read "与采配水交互全局.vi" "状态"() -> (w367:T3)
                n166 = Unbundle By Name(w367) -> ("R0"=w373:i16)
                n167 = Equal?(x=w373, y=i16 6) -> (x = y?=w371:bool)
                n168 = Select(t=enum16{"初始化", "采配水启动", "等待", "配水", "排水", "结束"}."配水" ("枚举"), s=w371, f=w369) -> (s? t:f=w368:enum16{"初始化", "采配水启动", "等待", "配水", "排水", "结束"})
              }
            }
          }
          frame "配水" {
            (unwired) cluster{"命令":string, "data":variant} {"命令"="启动", "data"=variant(cluster{"站号":u16, "控制命令输出":u16[]} {"站号"=1, "控制命令输出"=[256, 0]})} ("元素")
            n169 = Unbundle By Name(w391) -> ("是否启用仪器"=w393:bool, "启动模块.氨氮"=w389:bool, "启动模块.总磷"=w390:bool, "启动模块.总氮"=w387:bool, "启动模块.CODMn"=w388:bool, "启动模块.CODCr"=w386:bool)
            n170 = case shown="真" w393 {
              tunnel: w394 -> [_ w414]
              tunnel: [w398 w457] -> w392
              tunnel: w390 -> [_ w415]
              tunnel: w389 -> [_ w431]
              tunnel: w388 -> [_ w409]
              tunnel: w387 -> [_ w411]
              tunnel: w384 -> [_ w433]
              tunnel: w386 -> [_ w406]
              tunnel: w385 -> [_ w413]
              tunnel: w383 -> [_ w454]
              tunnel: w382 -> [_ w451]
              tunnel: w381 -> [_ w449]
              tunnel: w380 -> [_ w443]
              tunnel: w379 -> [_ w442]
              tunnel: [_ w441] -> w378
              tunnel: [_ w440] -> w377
              tunnel: [_ w439] -> w376
              tunnel: [_ w438] -> w375
              tunnel: [_ w437] -> w374
              frame False {
                n171 = feedback #4() -> (w402:i32)  [unwired: 1 in]
                n172 = Increment(x=w402) -> (x+1=w401:i32)
                n173 = First Call?() -> (First Call?: T/F=w403:bool)
                n174 = Select(t=0, s=w403, f=w401) -> (s? t:f=w399:i32)
                n175 = feedback-in #4(w399) -> ()
                n176 = Greater Or Equal?(x=w399, y=900) -> (x >= y?=w398:bool)
              }
              frame True {
                n177 = vi-ref "质控单元.lvlib:CODCr质控流程 (子VI).vi"() -> (w419:refnum<vi>)
                n178 = property class="VI"(reference=w419) -> ("Name"=w420:string, "Exec.State"=w418:T4)  [unwired: 1 in, 2 out]
                n179 = case shown="\"Idle\"" w418 {
                  tunnel: w420 -> [_ w464 _ _]
                  tunnel: [_ w459 _ _] -> w405
                  tunnel: w406 -> [_ w458 _ _]
                  frame "Bad", Default {
                  }
                  frame "Idle" {
                    n180 = First Call?() -> (First Call?: T/F=w463:bool)
                    n181 = case shown="真" w463 {
                      tunnel: w464 -> [_ w471]
                      tunnel: w458 -> [_ w465]
                      frame False {
                      }
                      frame True {
                        n182 = Open VI Reference(type specifier VI Refnum (for type only)=refnum<vi> refnum ("类型说明符VI引用句柄（仅用于类型）"), vi path=w471, options=128 ("选项")) -> (vi reference=w472:refnum<vi>, error out=w468:errorcluster)  [unwired: 3 in]
                        n183 = call-by-ref "开始异步调用"(reference=w472, error in=w468, "CODCr"=w465) -> (reference out=w470:refnum<vi>, error out=w469:errorcluster)  [unwired: 9 in, 1 out]
                        n184 = Close Reference(reference=w470, error in (no error)=w469) -> ()  [unwired: 1 out]
                      }
                    }
                    n185 = First Call?() -> (First Call?: T/F=w462:bool)
                    n186 = Select(t=FALSE, s=w462, f=TRUE) -> (s? t:f=w459:bool)
                  }
                  frame "Run top level" {
                  }
                  frame "Running" {
                  }
                }
                n187 = vi-ref "质控单元.lvlib:氨氮质控流程.vi"() -> (w435:refnum<vi>)
                n188 = vi-ref "质控单元.lvlib:总氮质控流程.vi"() -> (w425:refnum<vi>)
                n189 = vi-ref "质控单元.lvlib:总磷质控流程.vi"() -> (w428:refnum<vi>)
                n190 = property class="VI"(reference=w435) -> ("Name"=w434:string, "Exec.State"=w436:T4)  [unwired: 1 in, 2 out]
                n191 = property class="VI"(reference=w425) -> ("Name"=w426:string, "Exec.State"=w424:T4)  [unwired: 1 in, 2 out]
                n192 = property class="VI"(reference=w428) -> ("Name"=w427:string, "Exec.State"=w429:T4)  [unwired: 1 in, 2 out]
                n193 = local read "CODMn量程切换"() -> (w407:enum32{"H", "L", "AUTO"})
                n194 = case shown="\"Idle\"" w436 {
                  tunnel: w434 -> [_ w536 _ _]
                  tunnel: [_ w531 _ _] -> w430
                  tunnel: w433 -> [_ w530 _ _]
                  tunnel: "氨氮量程切换" -> [_ w529 _ _]
                  tunnel: w431 -> [_ w528 _ _]
                  frame "Bad", Default {
                  }
                  frame "Idle" {
                    n195 = First Call?() -> (First Call?: T/F=w535:bool)
                    n196 = case shown="真" w535 {
                      tunnel: w536 -> [_ w545]
                      tunnel: w530 -> [_ w539]
                      tunnel: w529 -> [_ w538]
                      tunnel: w528 -> [_ w537]
                      frame False {
                      }
                      frame True {
                        n197 = Open VI Reference(type specifier VI Refnum (for type only)=refnum<vi> refnum ("类型说明符VI引用句柄（仅用于类型）"), vi path=w545, options=128 ("选项")) -> (vi reference=w546:refnum<vi>, error out=w542:errorcluster)  [unwired: 3 in]
                        n198 = call-by-ref "开始异步调用"(reference=w546, error in=w542, "队列输入NH3"=w539, "氨氮"=w537, "氨氮量程切换"=w538) -> (reference out=w544:refnum<vi>, error out=w543:errorcluster)  [unwired: 7 in, 1 out]
                        n199 = Close Reference(reference=w544, error in (no error)=w543) -> ()  [unwired: 1 out]
                      }
                    }
                    n200 = First Call?() -> (First Call?: T/F=w534:bool)
                    n201 = Select(t=FALSE, s=w534, f=TRUE) -> (s? t:f=w531:bool)
                  }
                  frame "Run top level" {
                  }
                  frame "Running" {
                  }
                }
                n202 = case shown="\"Idle\"" w424 {
                  tunnel: w426 -> [_ w498 _ _]
                  tunnel: [_ w493 _ _] -> w410
                  tunnel: w413 -> [_ w492 _ _]
                  tunnel: "总氮量程切换" -> [_ w491 _ _]
                  tunnel: w411 -> [_ w490 _ _]
                  frame "Bad", Default {
                  }
                  frame "Idle" {
                    n203 = First Call?() -> (First Call?: T/F=w497:bool)
                    n204 = case shown="真" w497 {
                      tunnel: w498 -> [_ w508]
                      tunnel: w492 -> [_ w501]
                      tunnel: w491 -> [_ w500]
                      tunnel: w490 -> [_ w499]
                      frame False {
                      }
                      frame True {
                        n205 = Open VI Reference(type specifier VI Refnum (for type only)=refnum<vi> refnum ("类型说明符VI引用句柄（仅用于类型）"), vi path=w508, options=128 ("选项")) -> (vi reference=w503:refnum<vi>, error out=w502:errorcluster)  [unwired: 3 in]
                        n206 = call-by-ref "开始异步调用"(reference=w503, error in=w502, "队列输入TN"=w501, "总氮"=w499, "总氮量程切换"=w500) -> (reference out=w507:refnum<vi>, error out=w506:errorcluster)  [unwired: 7 in, 1 out]
                        n207 = Close Reference(reference=w507, error in (no error)=w506) -> ()  [unwired: 1 out]
                      }
                    }
                    n208 = First Call?() -> (First Call?: T/F=w496:bool)
                    n209 = Select(t=FALSE, s=w496, f=TRUE) -> (s? t:f=w493:bool)
                  }
                  frame "Run top level" {
                  }
                  frame "Running" {
                  }
                }
                n210 = case shown="\"Idle\"" w429 {
                  tunnel: w427 -> [_ w517 _ _]
                  tunnel: [_ w512 _ _] -> w416
                  tunnel: "总磷量程切换" -> [_ w511 _ _]
                  tunnel: w415 -> [_ w510 _ _]
                  tunnel: w414 -> [_ w509 _ _]
                  frame "Bad", Default {
                  }
                  frame "Idle" {
                    n211 = First Call?() -> (First Call?: T/F=w516:bool)
                    n212 = case shown="真" w516 {
                      tunnel: w517 -> [_ w518]
                      tunnel: w511 -> [_ w526]
                      tunnel: w510 -> [_ w524]
                      tunnel: w509 -> [_ w523]
                      frame False {
                      }
                      frame True {
                        n213 = Open VI Reference(type specifier VI Refnum (for type only)=refnum<vi> refnum ("类型说明符VI引用句柄（仅用于类型）"), vi path=w518, options=128 ("选项")) -> (vi reference=w522:refnum<vi>, error out=w521:errorcluster)  [unwired: 3 in]
                        n214 = call-by-ref "开始异步调用"(reference=w522, error in=w521, "队列输入TP"=w523, "总磷"=w524, "总磷量程切换"=w526) -> (reference out=w520:refnum<vi>, error out=w519:errorcluster)  [unwired: 7 in, 1 out]
                        n215 = Close Reference(reference=w520, error in (no error)=w519) -> ()  [unwired: 1 out]
                      }
                    }
                    n216 = First Call?() -> (First Call?: T/F=w515:bool)
                    n217 = Select(t=FALSE, s=w515, f=TRUE) -> (s? t:f=w512:bool)
                  }
                  frame "Run top level" {
                  }
                  frame "Running" {
                  }
                }
                n218 = vi-ref "质控单元.lvlib:CODMn质控流程 (子VI).vi"() -> (w422:refnum<vi>)
                n219 = property class="VI"(reference=w422) -> ("Name"=w421:string, "Exec.State"=w423:T4)  [unwired: 1 in, 2 out]
                n220 = case shown="\"Idle\"" w423 {
                  tunnel: w421 -> [_ w480 _ _]
                  tunnel: [_ w475 _ _] -> w408
                  tunnel: w409 -> [_ w474 _ _]
                  tunnel: w407 -> [_ w473 _ _]
                  frame "Bad", Default {
                  }
                  frame "Idle" {
                    n221 = First Call?() -> (First Call?: T/F=w479:bool)
                    n222 = case shown="真" w479 {
                      tunnel: w480 -> [_ w488]
                      tunnel: w474 -> [_ w482]
                      tunnel: w473 -> [_ w481]
                      frame False {
                      }
                      frame True {
                        n223 = Open VI Reference(type specifier VI Refnum (for type only)=refnum<vi> refnum ("类型说明符VI引用句柄（仅用于类型）"), vi path=w488, options=128 ("选项")) -> (vi reference=w489:refnum<vi>, error out=w485:errorcluster)  [unwired: 3 in]
                        n224 = call-by-ref "开始异步调用"(reference=w489, error in=w485, "CODMn量程切换"=w481, "CODMn"=w482) -> (reference out=w487:refnum<vi>, error out=w486:errorcluster)  [unwired: 8 in, 1 out]
                        n225 = Close Reference(reference=w487, error in (no error)=w486) -> ()  [unwired: 1 out]
                      }
                    }
                    n226 = First Call?() -> (First Call?: T/F=w478:bool)
                    n227 = Select(t=FALSE, s=w478, f=TRUE) -> (s? t:f=w475:bool)
                  }
                  frame "Run top level" {
                  }
                  frame "Running" {
                  }
                }
                n228 = Get Notifier Status(notifier=w442) -> (notifier out=w437:refnum<notifier>, current notification=w446:bool)  [unwired: 1 in, 3 out]
                n229 = Get Notifier Status(notifier=w443) -> (notifier out=w438:refnum<notifier>, current notification=w447:bool)  [unwired: 1 in, 3 out]
                n230 = Get Notifier Status(notifier=w449) -> (notifier out=w439:refnum<notifier>, current notification=w450:bool)  [unwired: 1 in, 3 out]
                n231 = Get Notifier Status(notifier=w451) -> (notifier out=w440:refnum<notifier>, current notification=w453:bool)  [unwired: 1 in, 3 out]
                n232 = Or(x=w405, y=w446) -> (x .or. y?=w444:bool)
                n233 = Or(x=w408, y=w447) -> (x .or. y?=w445:bool)
                n234 = Or(x=w410, y=w450) -> (x .or. y?=w448:bool)
                n235 = Get Notifier Status(notifier=w454) -> (notifier out=w441:refnum<notifier>, current notification=w456:bool)  [unwired: 1 in, 3 out]
                n236 = Or(x=w416, y=w453) -> (x .or. y?=w452:bool)
                n237 = Or(x=w430, y=w456) -> (x .or. y?=w455:bool)
                n238 = Compound Arithmetic op=AND ("复合运算")(w455, w452, w448, w445, w444) -> (w457:bool)
              }
            }
            n239 = Select(t=enum16{"初始化", "采配水启动", "等待", "配水", "排水", "结束"}."排水" ("枚举"), s=w392, f=w396) -> (s? t:f=w395:enum16{"初始化", "采配水启动", "等待", "配水", "排水", "结束"})
          }
          frame "排水" {
            n240 = Enqueue Element At Opposite End(queue=w549, element=T2 {"命令"="单个写入", {"starting address"=303, "holding register value"=1}} ("元素")) -> ()  [unwired: 2 in, 3 out]
            n241 = Increment(x=w548) -> (x+1=w547:enum16{"初始化", "采配水启动", "等待", "配水", "排水", "结束"})
          }
          frame "结束" {
            n242 = Increment(x=w553) -> (x+1=w552:enum16{"初始化", "采配水启动", "等待", "配水", "排水", "结束"})
          }
        }
        "枚举" <- w347
        n243 = Wait (ms)(milliseconds to wait=u32 1000 ("等待时间（毫秒）")) -> ()  [unwired: 1 out]
        n244 = global write "质控测完标志全局 1.vi" "质控流程中"(TRUE ("质控流程中")) -> ()
        n245 = Get Notifier Status(notifier=w343) -> (notifier out=w342:refnum<notifier>, current notification=w340:bool)  [unwired: 1 in, 3 out]
        n246 = Or(x=w340, y=w341) -> (x .or. y?=w339:bool)
        n247 = case shown="真" w339 {
          frame False {
          }
          frame True {
            w350 = FALSE ("质控流程中")
            n248 = global write "质控测完标志全局 1.vi" "质控流程中"(w350) -> ()
            n249 = global write "质控测完标志全局 1.vi" "COD加标回收测完标志"(w350) -> ()
            n250 = global write "质控测完标志全局 1.vi" "总氮加标回收测完标志"(w350) -> ()
            n251 = global write "质控测完标志全局 1.vi" "氨氮加标回收测完标志"(w350) -> ()
            n252 = global write "质控测完标志全局 1.vi" "CODCr加标回收测完标志"(w350) -> ()
            n253 = global write "质控测完标志全局 1.vi" "总磷加标回收测完标志"(w350) -> ()
          }
        }
      }
      n254 = Cancel Notification(0:w282) -> (8:w283:refnum<notifier>)  [unwired: 1 in, 2 out]
      n255 = Cancel Notification(0:w284) -> (8:w285:refnum<notifier>)  [unwired: 1 in, 2 out]
      n256 = Cancel Notification(0:w286) -> (8:w287:refnum<notifier>)  [unwired: 1 in, 2 out]
      n257 = Cancel Notification(0:w288) -> (8:w289:refnum<notifier>)  [unwired: 1 in, 2 out]
      n258 = Cancel Notification(0:w290) -> (8:w291:refnum<notifier>)  [unwired: 1 in, 2 out]
      n259 = Cancel Notification(0:w315) -> (8:w314:refnum<notifier>)  [unwired: 1 in, 2 out]
      n260 = Release Notifier(notifier=w283) -> ()  [unwired: 2 in, 3 out]
      n261 = Release Notifier(notifier=w285) -> ()  [unwired: 2 in, 3 out]
      n262 = Release Notifier(notifier=w287) -> ()  [unwired: 2 in, 3 out]
      n263 = Release Notifier(notifier=w289) -> ()  [unwired: 2 in, 3 out]
      n264 = Release Notifier(notifier=w291) -> ()  [unwired: 2 in, 3 out]
      n265 = Release Notifier(notifier=w314) -> ()  [unwired: 2 in, 3 out]
    }
  }
